vi "RichToFlatcif_plugincore_Configuration.vi"(5 "OutputClusterType":T1, 11 "InputCluster":T2) -> (3 "OutputCluster":T1)   [LabVIEW 2021, in "CIFCorePlugin_client.lvlib"]
uses:
  CIFCorePlugin_client.lvlib
  cif_plugincore_Configuration.ctl
  cif_plugincore_Configuration_Flat.ctl
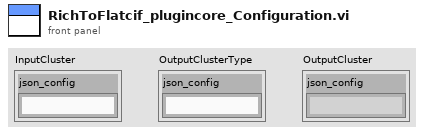
[diagram p1: front panel]
types:
  T1 = typedef "CIFCorePlugin_client.lvlib/cif_plugincore_Configuration_Flat.ctl" = cluster{"json_config":string}
  T2 = typedef "CIFCorePlugin_client.lvlib/cif_plugincore_Configuration.ctl" = cluster{"json_config":string}
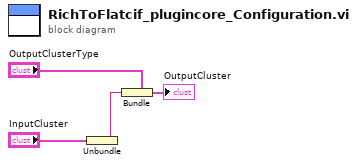
[diagram p0: block diagram]
diagram:
  n1 = Unbundle "Unbundle"("InputCluster") -> ("json_config"=w1:string)
  n2 = Bundle "Bundle"(cluster="OutputClusterType", "json_config"=w1) -> (→"OutputCluster":T1)
